vi "Test 2d axis control.vi"() -> ()   [LabVIEW 2012]
uses:
  Reusable/Xctls/Buffer/2D Control/2D Buffer Display.xctl
panel:
  in  "Boolean":bool
  out "2D Buffer Display":cluster{"data_out":sgl[][], "time":timestamp}(xcontrol)
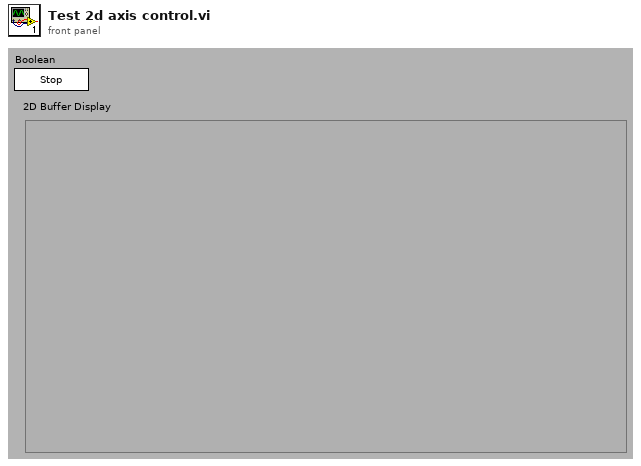
[diagram p1: front panel]
types:
  T1 = cluster{"Name":string, "Line Width":u8, "Line Style":u8, "Color":u32}[]
  T2 = cluster{dbl[][], "seconds since 1Jan1904":timestamp}
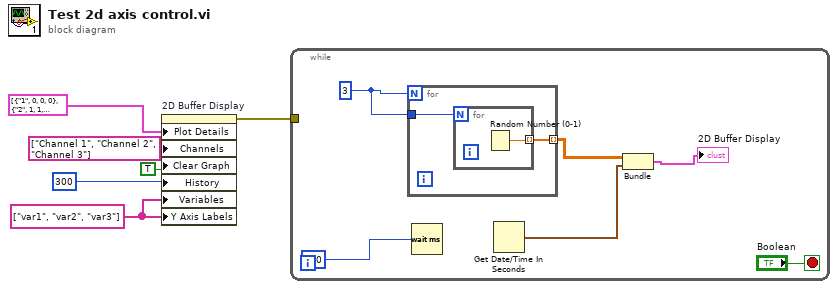
[diagram p0: block diagram]
diagram:
  w3 = string[] ["var1", "var2", "var3"] ("Y Axis Labels")
  n1 = property on="2D Buffer Display" class="2D Buffer Display (strict)"("Plot Details"=T1 [{"Name"="1", "Line Width"=0, "Line Style"=0, "Color"=0}, {"Name"="2", "Line Width"=1, "Line Style"=1, "Color"=16860}, {"Name"="3", "Line Width"=1, "Line Style"=1, "Color"=16711680}], "Channels"=string[] ["Channel 1", "Channel 2", "Channel 3"], "Clear Graph"=TRUE, "History"=u16 300, "Variables"=w3, "Y Axis Labels"=w3) -> (error out=w1:errorcluster)  [unwired: 2 in, 1 out]
  n2 = while {
    tunnel: w1 -> [_]
    stop <- "Boolean" stop-if-true
    w8 = 3
    n3 = for {
      N: w8 -> [_]
      tunnel: [w14] -> w11 mode=indexing
      tunnel: w8 -> [w13]
      n4 = for {
        N: w13 -> [_]
        tunnel: [w15] -> w14 mode=indexing
        n5 = Random Number (0-1)() -> (number: 0 to 1=w15:dbl)
      }
    }
    n6 = Wait (ms)(milliseconds to wait=u32 100) -> ()  [unwired: 1 out]
    n7 = Get Date/Time In Seconds() -> (seconds since 1Jan1904=w10:timestamp)
    n8 = Bundle(w11, "seconds since 1Jan1904"=w10) -> (→"2D Buffer Display":T2)  [unwired: 1 in]
  }
